vi "class names FGV.vi"(5 "class type":T1, 7 "Action":T3=enum."Write Type", 10 "class metadata":T2, 11 "classes info in":T2[](array[typedef])) -> (3 "classes info out":T2[](array[typedef]))   [LabVIEW 2013, in "PL_class cache.lvlib"]
uses:
  PL_class cache.lvlib
  class FGV actions.ctl
  class metadata.ctl
  class type.ctl
  class FGV data.ctl
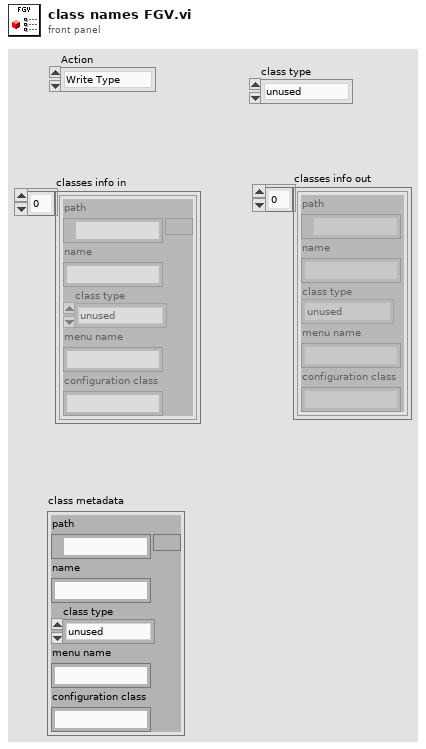
[diagram p1: front panel]
types:
  T1 = typedef "PL_class cache.lvlib/class type.ctl" = enum16{"unused", "other pl", "system", "target", "engine", "module"}
  T2 = typedef "PL_class cache.lvlib/class metadata.ctl" = cluster{"path":path, "name":string, "class type":T1, "menu name":string, "configuration class":string}
  T3 = typedef "PL_class cache.lvlib/class FGV actions.ctl" = enum16{"Add Element to Type", "Write Type", "Read  Type", "Read All", "Init"}
  T4 = typedef "PL_class cache.lvlib/class FGV data.ctl" = cluster{"modules":T2[], "Engines":T2[], "Targets":T2[], "Other":T2[]}
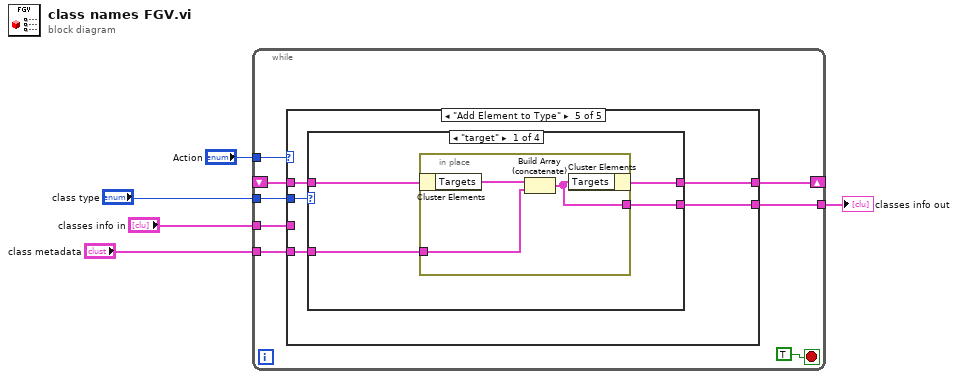
[diagram p0: block diagram]
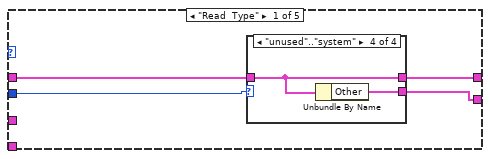
[diagram p2: hidden frame]
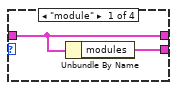
[diagram p3: hidden frame]
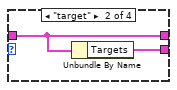
[diagram p4: hidden frame]
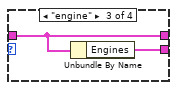
[diagram p5: hidden frame]
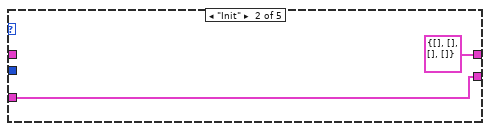
[diagram p6: hidden frame]
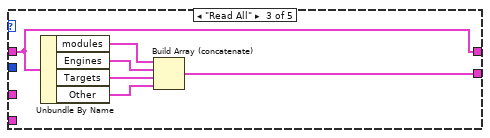
[diagram p7: hidden frame]
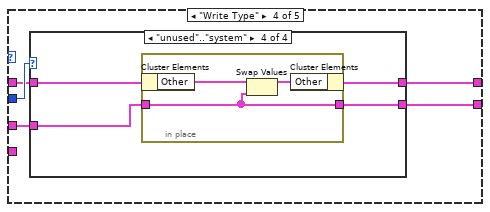
[diagram p8: hidden frame]
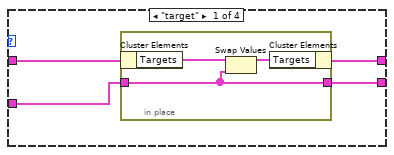
[diagram p9: hidden frame]
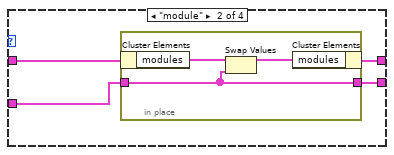
[diagram p10: hidden frame]
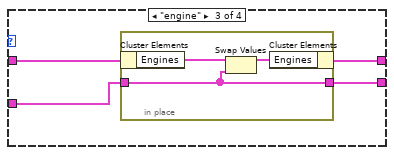
[diagram p11: hidden frame]
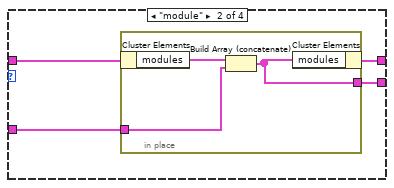
[diagram p12: hidden frame]
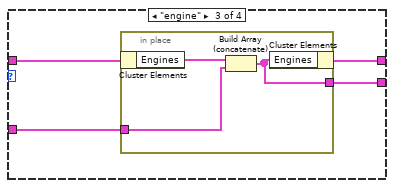
[diagram p13: hidden frame]
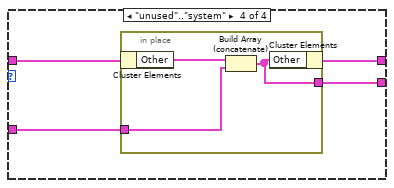
[diagram p14: hidden frame]
diagram:
  n1 = while {
    shift-right: [w11] -> _
    shift-left: _ -> [w12]
    tunnel: "Action" -> [w10]
    tunnel: "class type" -> [w9]
    tunnel: "classes info in" -> [w8]
    tunnel: [w7] -> w3
    tunnel: "class metadata" -> [w6]
    stop <- TRUE ("stop") stop-if-true
    n2 = case shown="\"Add Element to Type\"" w10 {
      tunnel: w12 -> [w17 _ w33 w37 w70]
      tunnel: [w16 T4 {"modules"=[], "Engines"=[], "Targets"=[], "Other"=[]} ("Class Names FGV Data") w33 w36 w69] -> w11
      tunnel: w9 -> [w15 _ _ w38 w71]
      tunnel: w8 -> [_ w26 _ w35 _]
      tunnel: [w14 w26 w28 w34 w68] -> w7
      tunnel: w6 -> [_ _ _ _ w67]
      frame "Read  Type" {
        n3 = case shown="\"unused\"..\"system\"" w15 {
          tunnel: w17 -> [w19 w21 w23 w25]
          tunnel: [w19 w21 w23 w25] -> w16
          tunnel: [w18 w20 w22 w24] -> w14
          frame "module" {
            n4 = Unbundle By Name(w19) -> ("modules"=w18:T2[])
          }
          frame "target" {
            n5 = Unbundle By Name(w21) -> ("Targets"=w20:T2[])
          }
          frame "engine" {
            n6 = Unbundle By Name(w23) -> ("Engines"=w22:T2[])
          }
          frame "unused".."system" {
            n7 = Unbundle By Name(w25) -> ("Other"=w24:T2[])
          }
        }
      }
      frame "Init" {
      }
      frame "Read All" {
        n8 = Unbundle By Name(w33) -> ("modules"=w32:T2[], "Engines"=w31:T2[], "Targets"=w30:T2[], "Other"=w29:T2[])
        n9 = Build Array (concatenate)(w32, w31, w30, w29) -> (w28:T2[])
      }
      frame "Write Type" {
        n10 = case shown="\"unused\"..\"system\"" w38 {
          tunnel: w37 -> [w42 w49 w56 w63]
          tunnel: [w41 w48 w55 w62] -> w36
          tunnel: w35 -> [w40 w47 w54 w61]
          tunnel: [w39 w46 w53 w60] -> w34
          frame "target" {
            n11 = in-place {
              in-place-border: w40 -> [w43]
              in-place-border: [w43] -> w39
              n12 = in-place-cluster #1(w42) -> ("Targets"=w45:T2[])
              n13 = Swap Values(12:w45, 14:w43) -> (1:w44:T2[])  [unwired: 1 in, 1 out]
              n14 = in-place-cluster #1("Targets"=w44) -> (w41:T4)
            }
          }
          frame "module" {
            n15 = in-place {
              in-place-border: w47 -> [w50]
              in-place-border: [w50] -> w46
              n16 = in-place-cluster #2(w49) -> ("modules"=w52:T2[])
              n17 = Swap Values(12:w52, 14:w50) -> (1:w51:T2[])  [unwired: 1 in, 1 out]
              n18 = in-place-cluster #2("modules"=w51) -> (w48:T4)
            }
          }
          frame "engine" {
            n19 = in-place {
              in-place-border: w54 -> [w57]
              in-place-border: [w57] -> w53
              n20 = in-place-cluster #3(w56) -> ("Engines"=w59:T2[])
              n21 = Swap Values(12:w59, 14:w57) -> (1:w58:T2[])  [unwired: 1 in, 1 out]
              n22 = in-place-cluster #3("Engines"=w58) -> (w55:T4)
            }
          }
          frame "unused".."system" {
            n23 = in-place {
              in-place-border: w61 -> [w64]
              in-place-border: [w64] -> w60
              n24 = in-place-cluster #4(w63) -> ("Other"=w66:T2[])
              n25 = Swap Values(12:w66, 14:w64) -> (1:w65:T2[])  [unwired: 1 in, 1 out]
              n26 = in-place-cluster #4("Other"=w65) -> (w62:T4)
            }
          }
        }
      }
      frame "Add Element to Type" {
        n27 = case shown="\"target\"" w71 {
          tunnel: w70 -> [w75 w82 w89 w96]
          tunnel: [w74 w81 w88 w95] -> w69
          tunnel: [w72 w80 w86 w94] -> w68
          tunnel: w67 -> [w73 w79 w87 w93]
          frame "target" {
            n28 = in-place {
              in-place-border: w73 -> [w77]
              in-place-border: [w76] -> w72
              n29 = in-place-cluster #5(w75) -> ("Targets"=w78:T2[])
              n30 = Build Array (concatenate)(w78, w77) -> (w76:T2[])
              n31 = in-place-cluster #5("Targets"=w76) -> (w74:T4)
            }
          }
          frame "module" {
            n32 = in-place {
              in-place-border: [w84] -> w80
              in-place-border: w79 -> [w83]
              n33 = in-place-cluster #6(w82) -> ("modules"=w85:T2[])
              n34 = Build Array (concatenate)(w85, w83) -> (w84:T2[])
              n35 = in-place-cluster #6("modules"=w84) -> (w81:T4)
            }
          }
          frame "engine" {
            n36 = in-place {
              in-place-border: w87 -> [w91]
              in-place-border: [w90] -> w86
              n37 = in-place-cluster #7(w89) -> ("Engines"=w92:T2[])
              n38 = Build Array (concatenate)(w92, w91) -> (w90:T2[])
              n39 = in-place-cluster #7("Engines"=w90) -> (w88:T4)
            }
          }
          frame "unused".."system" {
            n40 = in-place {
              in-place-border: [w98] -> w94
              in-place-border: w93 -> [w97]
              n41 = in-place-cluster #8(w96) -> ("Other"=w99:T2[])
              n42 = Build Array (concatenate)(w99, w97) -> (w98:T2[])
              n43 = in-place-cluster #8("Other"=w98) -> (w95:T4)
            }
          }
        }
      }
    }
  }
  "classes info out" <- w3
